vi "EditQTrkSettingsDialog.vi"(10 "ROI":i32, 11 "Settings":T2={"Image width"=100, "Image height"=100, "Number of threads (CPU based)"=-1, "CUDA Device"=-2, "COM Background correction factor"=0.0, "ZLUT MinRadius"=3.0, "ZLUT Radial sample density"=2.0, "ZLUT Angular sample density"=0.7, "ZLUT ROI Coverage"=1.0, "QI Iterations"=5, "QI MinRadius"=5.0, "QI Radial sample density"=2.0, "QI Angular sample density"=0.7, "QI ROI Coverage"=1.0, "QI Angular Step \nIteration Factor"=1.0, "XCOR Profile Length"=128, "XCOR Profile Width"=32, "XCOR Iterations"=2, "Gaussian 2D Fit Iterations"=6, "Gaussian 2D Sigma (pixels)"=3.0, "Downsample"=0} {"QI Angular Step \nIteration Factor" format="%_3g"; "COM Background correction factor" format="%.2f"; "QI ROI Coverage" format="%.2g"; "QI Angular sample density" format="%.2f"; "QI Radial sample density" format="%.2f"; "ZLUT Radial sample density" format="%.2f"}) -> (3 "Settings (output)":T2={"Image width"=150, "Image height"=150, "Number of threads (CPU based)"=-1, "CUDA Device"=200, "COM Background correction factor"=128.0, "ZLUT MinRadius"=32.0, "ZLUT Radial sample density"=2.0, "ZLUT Angular sample density"=5.0, "ZLUT ROI Coverage"=50.0, "QI Iterations"=64, "QI MinRadius"=4.0, "QI Radial sample density"=64.0, "QI Angular sample density"=64.0, "QI ROI Coverage"=2.0, "QI Angular Step \nIteration Factor"=50.0, "XCOR Profile Length"=0, "XCOR Profile Width"=2, "XCOR Iterations"=32, "Gaussian 2D Fit Iterations"=8, "Gaussian 2D Sigma (pixels)"=3.0, "Downsample"=0})   [LabVIEW 2011]
uses:
  qtrk/QTrkLVBinding/QTrkSettings.ctl
  qtrk/QTrkLVBinding/QTrkLocalizationType.ctl
panel:
  in  "Z Localization?":bool=TRUE
  in  "Speed test mode:":T1=enum."Quadrant Interpolation"
  out "Images/s:":dbl
  in  "Speed test":bool
  in  "OK":bool
  # "-2: Use all devices\n-1: Use best device"
  # "-2: Use all devices\n-1: Use best device"
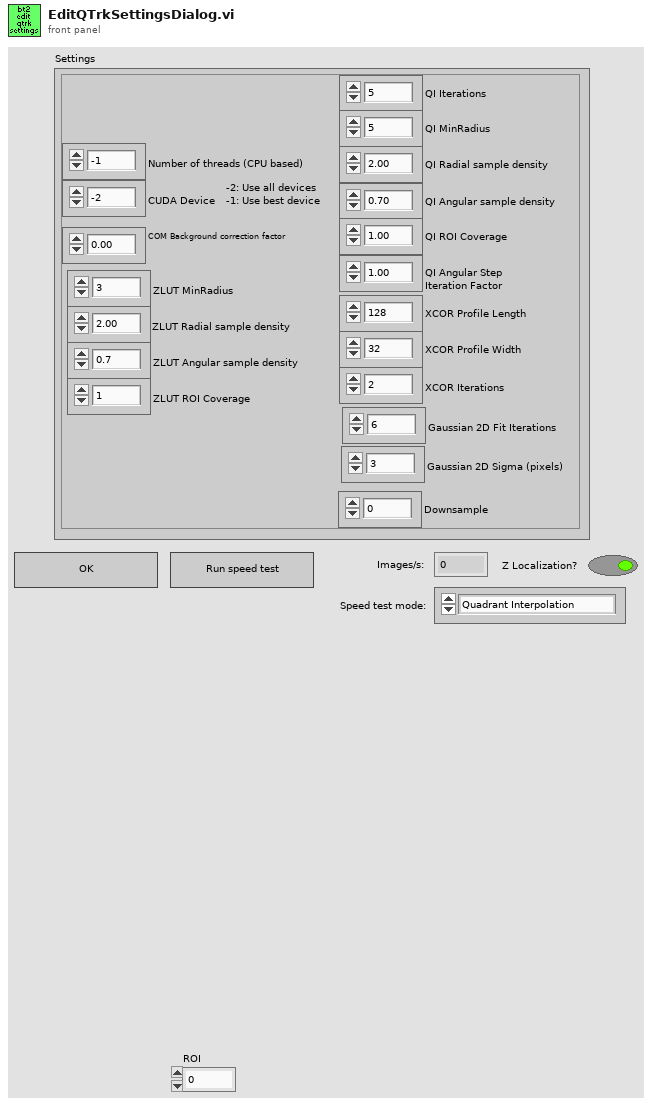
[diagram p1: front panel]
types:
  T1 = typedef "QTrkLocalizationType.ctl" = enum16{"Center-of-Mass", "1D Cross-Correlation", "Quadrant Interpolation", "Gaussian 2D MLE", "QI + ZLUTAlign", "ZLUTAlign", "QI + FourierLUT"}
  T2 = typedef "QTrkSettings.ctl" = cluster{"Image width":i32, "Image height":i32, "Number of threads (CPU based)":i32, "CUDA Device":i32, "COM Background correction factor":sgl, "ZLUT MinRadius":sgl, "ZLUT Radial sample density":sgl, "ZLUT Angular sample density":sgl, "ZLUT ROI Coverage":sgl, "QI Iterations":i32, "QI MinRadius":sgl, "QI Radial sample density":sgl, "QI Angular sample density":sgl, "QI ROI Coverage":sgl, "QI Angular Step \nIteration Factor":sgl, "XCOR Profile Length":i32, "XCOR Profile Width":i32, "XCOR Iterations":i32, "Gaussian 2D Fit Iterations":i32, "Gaussian 2D Sigma (pixels)":sgl, "Downsample":i32}
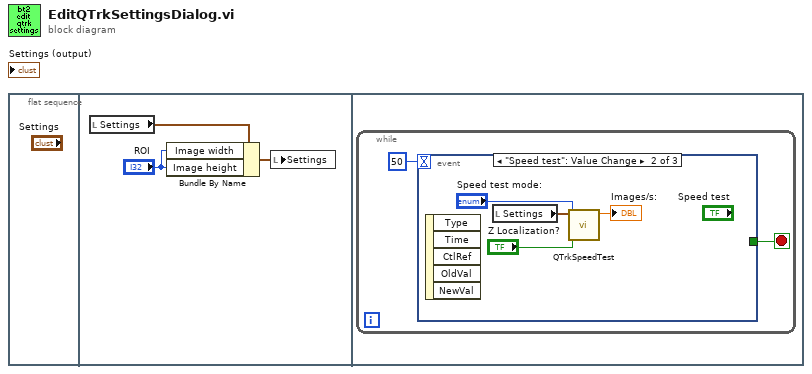
[diagram p0: block diagram]
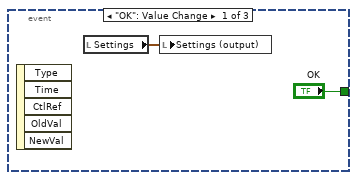
[diagram p2: hidden frame]
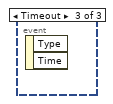
[diagram p3: hidden frame]
diagram:
  n1 = flat-sequence {
    frame #0 {
    }
    frame #1 {
      n2 = local read "Settings"() -> (w3:T2)
      n3 = Bundle By Name(cluster=w3, "Image width"="ROI", "Image height"="ROI") -> (w1:T2)
      n4 = local write "Settings"(w1) -> ()
    }
    frame #2 {
      n5 = while {
        stop <- w5 stop-if-true
        n6 = event shown="[1] \"Speed test\": Value Change" {
          selector: _ -> [_ _ _]
          dyn-events: _ -> [_ _ _]
          timeout: 50 -> [_ _ _]
          tunnel: ["OK" _ _] -> w5
          event "OK": Value Change {
            n7 = event-data() -> ()  [unwired: 1 in, 5 out]
            n8 = local read "Settings"() -> (w6:T2)
            n9 = local write "Settings (output)"(w6) -> ()
          }
          event "Speed test": Value Change {
            n10 = event-data() -> ()  [unwired: 1 in, 5 out]
            n11 = local read "Settings"() -> (w11:T2)
            n12 = call "QTrkSpeedTest.vi"("2D Localization Type"="Speed test mode:", "Z Localization?"="Z Localization?", "QTrk Settings"=w11) -> ("Images/s"=→"Images/s:":dbl)  [unwired: 7 in, 1 out]
          }
          event Timeout {
            n13 = event-data() -> ()  [unwired: 1 in, 2 out]
          }
        }
      }
    }
  }
